vi "Pre Launch Init.vi"(11 "Nested in":refnum<class "DisplayerUI.lvclass">) -> (0 "error out":errorcluster, 3 "Nested out":refnum<class "DisplayerUI.lvclass">)   [LabVIEW 2020, in "DisplayerUI.lvlib" / "DisplayerUI.lvclass"]
doc: "(<B>Filename</B>: Actor Framework.lvlib:Actor.lvclass:Pre Launch Init.vi)\n\nDefines behavior that occurs after the Launch Nested Actor method is invoked but before the actor's Actor Core method begins running.\n\nBy default, this method does nothing. A descendant class may override it to define behavior."
uses:
  DisplayerUI.lvclass
  <vilib>/vision/Image Controls.llb/IMAQ Image.ctl
  DisplayerUI.lvclass/DisplayerUI.ctl
  Hardware Abstraction Layer/Component/GenericActor/GenericActor/GenericController.lvclass
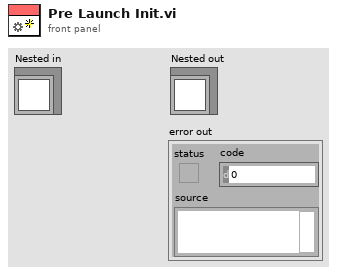
[diagram p1: front panel]
types:
  T1 = typedef "Image Type" = u32
  T2 = typedef "IMAQ Image.ctl" = refnum<image>
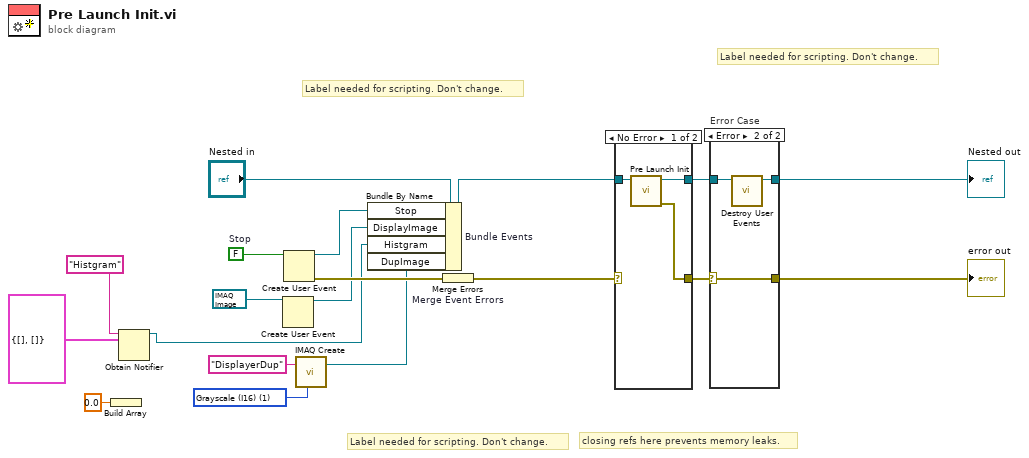
[diagram p0: block diagram]
diagram:
  w5 = T1 1 items=["Grayscale (U8)", "Grayscale (I16)", "Grayscale (SGL)", "Complex (CSG)", "RGB (U32)", "HSL (U32)", "RGB (U64)", "Grayscale (U16)"] ("Image Type")
  w18 = FALSE  # Stop
  # "Label needed for scripting. Don't change."
  # "Label needed for scripting. Don't change."
  # "Label needed for scripting. Don't change."
  # "closing refs here prevents memory leaks."
  n1 = Build Array(0.0 ("element")) -> ()  [unwired: 1 out]
  n2 = Obtain Notifier(name (unnamed)="Histgram", notification data type=cluster{"Histgram":dbl[], "Profile":dbl[]} {"Histgram"=[], "Profile"=[]}) -> (notifier out=w1:refnum<notifier>)  [unwired: 2 in, 2 out]
  n3 = Create User Event(user event datatype=T2 refnum ("RawImage")) -> (user event=w8:refnum<user-event>)  [unwired: 1 in, 1 out]
  n4 = Create User Event(user event datatype=w18) -> (user event=w15:refnum<user-event>, error out=w17:errorcluster)  [unwired: 1 in]
  n5 = call "IMAQ Create"("Image Name"="DisplayerDup", "Image Type"=w5) -> ("New Image"=w6:T2)  [unwired: 3 in, 1 out]
  n6 = Bundle By Name "Bundle Events"(cluster="Nested in", "Stop"=w15, "DisplayImage"=w8, "Histgram"=w1, "DupImage"=w6) -> (w12:refnum<class "DisplayerUI.lvclass">)
  n7 = Merge Errors "Merge Event Errors"(w17) -> (w11:errorcluster)
  n8 = case shown="No Error" w11 {
    selector: w11 -> [_ w24]
    tunnel: [w22 w23] -> w13
    tunnel: w12 -> [w21 w23]
    tunnel: [w20 w24] -> w10
    frame No Error {
      n9 = call-parent "Pre Launch Init.vi"("GenericController in"=w21) -> ("error out"=w20:errorcluster, "GenericController out"=w22:refnum<class "DisplayerUI.lvclass">)  [unwired: 9 in]
    }
    frame Error {
    }
  }
  n10 = case "Error Case" shown="Error" w10 {
    selector: w10 -> [w25 w29]
    tunnel: w13 -> [w26 w28]
    tunnel: [w26 w27] -> w16
    tunnel: [w25 w29] -> w14
    frame No Error {
    }
    frame Error {
      n11 = call "Destroy User Events.vi"("UI Template in"=w28) -> ("UI Template out"=w27:refnum<class "DisplayerUI.lvclass">)  [unwired: 10 in]
    }
  }
  "error out" <- w14
  "Nested out" <- w16
